vi "Send Log Data.vi"(8 "error in (no error)":errorcluster, 10 "Data":T1[](array[typedef]), 11 "Word Log Producer in":refnum<class "Word Log Producer.lvclass">) -> (0 "error out":errorcluster, 3 "Word Log Producer out":refnum<class "Word Log Producer.lvclass">)   [LabVIEW 2020, in "Ballard ARINC 429 Engine.lvlib" / "Implementation.lvlib" / "Word Logging.lvlib" / "Word Log Producer.lvclass"]
uses:
  Word Log Producer.lvclass
  Word.ctl
  Log Word Message/Log Word Message.lvclass
  C:/Program Files (x86)/National Instruments/LabVIEW 2020/vi.lib/NI/Messaging/Message/Abstract Message/Abstract Message.lvclass
  Word Log Producer.lvclass/Word Log Producer.ctl
  Word Logging.lvlib
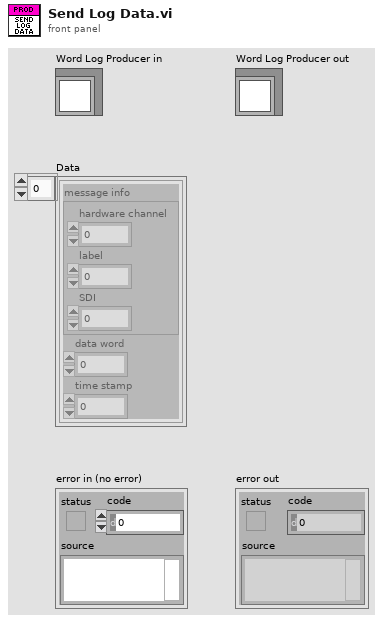
[diagram p1: front panel]
types:
  T1 = typedef "Ballard ARINC 429 Engine.lvlib/Implementation.lvlib/Word Logging.lvlib/Word.ctl" = cluster{"message info":cluster{"hardware channel":u8, "label":u8, "SDI":u8}, "data word":u32, "time stamp":dbl}
  T2 = typedef "Ballard ARINC 429 Engine.lvlib/Implementation.lvlib/Word Logging.lvlib/Word Logger Data Reference.ctl" = refnum<data-value>
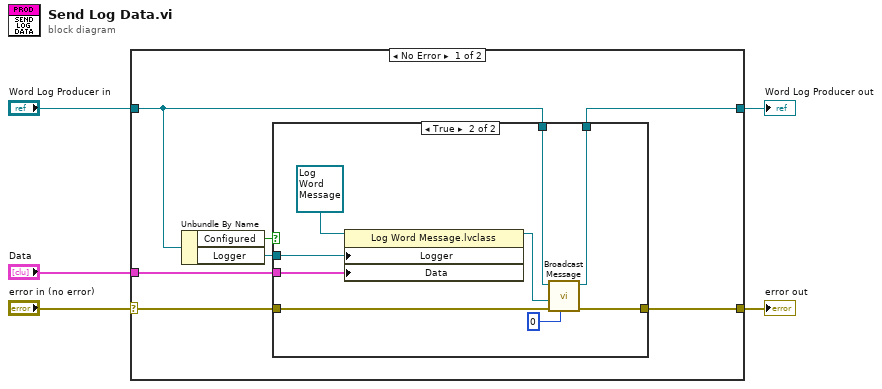
[diagram p0: block diagram]
diagram:
  n1 = case shown="No Error" "error in (no error)" {
    selector: "error in (no error)" -> [w11 w25]
    tunnel: [w10 w25] -> w4
    tunnel: [w8 w24] -> w2
    tunnel: "Word Log Producer in" -> [w9 w24]
    tunnel: "Data" -> [w7 _]
    frame No Error {
      n2 = Unbundle By Name(w9) -> ("Configured"=w6:bool, "Logger"=w12:T2)
      n3 = case shown="True" w6 {
        tunnel: w12 -> [_ w23]
        tunnel: w11 -> [w13 w22]
        tunnel: [w13 w21] -> w10
        tunnel: w9 -> [w14 w20]
        tunnel: [w14 w19] -> w8
        tunnel: w7 -> [_ w16]
        frame False {
        }
        frame True {
          n4 = property class="Log Word Message.lvclass"(reference=refnum<class "Log Word Message.lvclass"> refnum ("Communication Bus Template Interfaces:Implementation.lvlib:Logging.lvlib:Log Word Message.lvclass"), "Logger"=w23, "Data"=w16) -> (reference out=w18:refnum<class "Log Word Message.lvclass">)  [unwired: 1 in, 1 out]
          n5 = call-dynamic "Broadcast Message.vi"("timeout in ms (-1)"=0, "error in (no error)"=w22, "Message in"=w18, "Abstract Producer in"=w20) -> ("error out"=w21:errorcluster, "Abstract Producer out"=w19:refnum<class "Word Log Producer.lvclass">)  [unwired: 4 in, 2 out]
        }
      }
    }
    frame Error {
    }
  }
  "error out" <- w4
  "Word Log Producer out" <- w2
